vi "Set Status Event.vi"(8 "error in (no error)":errorcluster, 11 "hStatusEvent":u32) -> (0 "error out":errorcluster, 2 "function return":i32, 3 "hStatusEvent out":u32)   [LabVIEW 2020, in "ThorConfocal.lvlib"]
doc: "long SetStatusEvent(HANDLE hStatusEvent);"
uses:
  ThorConfocal.lvlib
  ThorConfocal.dll
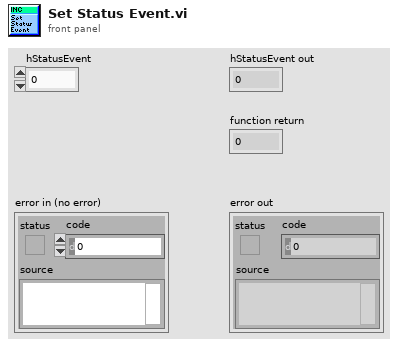
[diagram p1: front panel]
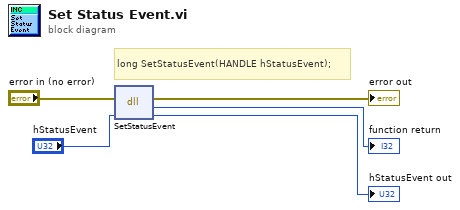
[diagram p0: block diagram]
diagram:
  # "long SetStatusEvent(HANDLE hStatusEvent);"
  n1 = dll-call lib="D:/software/TweezerTron/ThorConfocal.*" fn="SetStatusEvent"(error in="error in (no error)", "hStatusEvent"="hStatusEvent") -> (error out=→"error out":errorcluster, →"function return":i32, "hStatusEvent"=→"hStatusEvent out":u32)  [unwired: 2 in, 1 out]
